vi "Initialize.vi"(8 "error in (no error)":errorcluster) -> (0 "error out":errorcluster, 3 "Available motors out":refnum<class "Motor-assembly.lvclass">)   [LabVIEW 2013, in "PowderDeposition.lvlib" / "Motor-assembly.lvclass"]
doc: "Create all motor objects and set the default settings contained in the 'Create' override of each specific motor class."
uses:
  Motor-assembly.lvclass
  Motor/Motor-Serial/Motor-Maxon/Motor-Zaxis/Motor-Zaxis.lvclass
  Motor/Motor-Serial/Motor-Maxon/Motor-Xaxis/Motor-Xaxis.lvclass
  Motor/Motor-Serial/Motor-GWInstek/Motor-Roller2/Motor-Roller2.lvclass
  Motor/Motor-Serial/Motor-GWInstek/Motor-Sieve2/Motor-Sieve2.lvclass
  Motor-assembly.lvclass/Motor-assembly.ctl
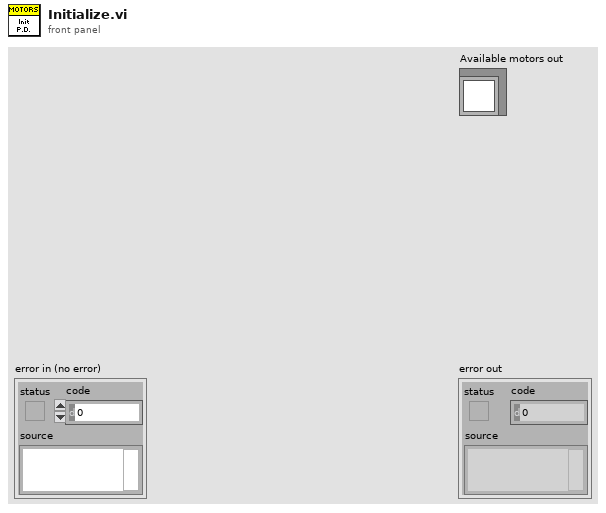
[diagram p1: front panel]
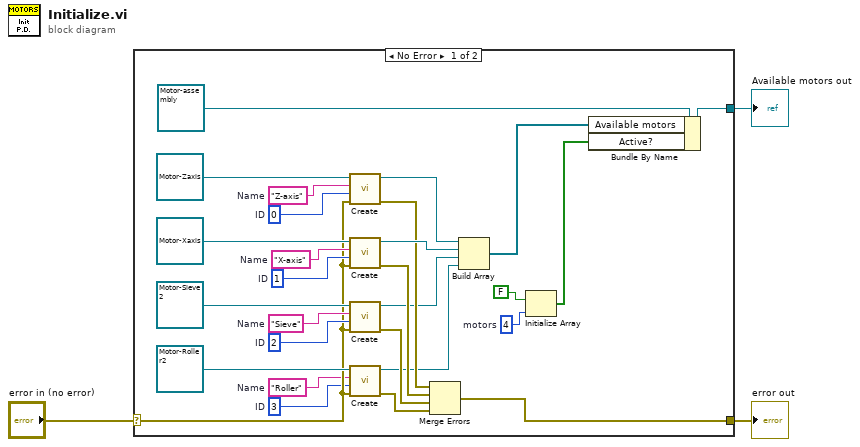
[diagram p0: block diagram]
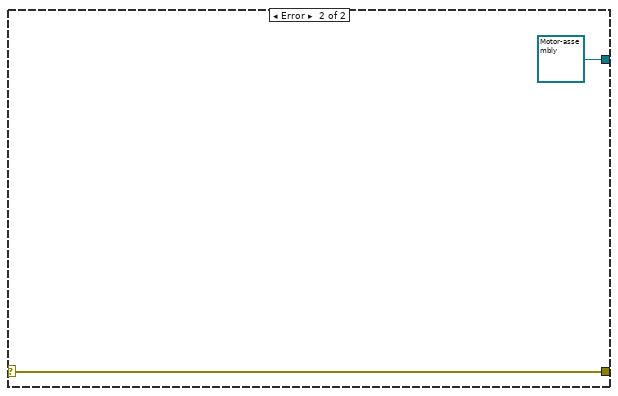
[diagram p2: hidden frame]
diagram:
  n1 = case shown="No Error" "error in (no error)" {
    selector: "error in (no error)" -> [w6 w33]
    tunnel: [w15 w33] -> w2
    tunnel: [w30 refnum<class "Motor-assembly.lvclass"> refnum ("Available motors in")] -> w1
    frame No Error {
      w20 = 4  # motors
      w5 = 3  # ID
      w4 = "Roller"  # Name
      w12 = 2  # ID
      w13 = "Sieve"  # Name
      w24 = 1  # ID
      w25 = "X-axis"  # Name
      w26 = 0  # ID
      w27 = "Z-axis"  # Name
      n2 = call-dynamic "Create.vi"("error in (no error)"=w6, "ID"=w26, "Name"=w27, "Motor in"=refnum<class "Motor-Zaxis.lvclass"> refnum ("Motor-Zaxis.lvclass")) -> ("error out"=w17:errorcluster, "Motor out"=w23:refnum<class "Motor-Zaxis.lvclass">)  [unwired: 6 in]
      n3 = call-dynamic "Create.vi"("error in (no error)"=w6, "ID"=w24, "Name"=w25, "Motor in"=refnum<class "Motor-Xaxis.lvclass"> refnum ("Motor-Xaxis.lvclass")) -> ("error out"=w16:errorcluster, "Motor out"=w22:refnum<class "Motor-Xaxis.lvclass">)  [unwired: 6 in]
      n4 = call-dynamic "Create.vi"("error in (no error)"=w6, "ID"=w12, "Name"=w13, "Motor in"=refnum<class "Motor-Sieve2.lvclass"> refnum ("Motor-Sieve2.lvclass")) -> ("error out"=w11:errorcluster, "Motor out"=w10:refnum<class "Motor-Sieve2.lvclass">)  [unwired: 6 in]
      n5 = call-dynamic "Create.vi"("error in (no error)"=w6, "ID"=w5, "Name"=w4, "Motor in"=refnum<class "Motor-Roller2.lvclass"> refnum ("Motor-Roller2.lvclass")) -> ("error out"=w7:errorcluster, "Motor out"=w8:refnum<class "Motor-Roller2.lvclass">)  [unwired: 6 in]
      n6 = Merge Errors(w17, w16, w11, w7) -> (w15:errorcluster)
      n7 = Build Array(w23, w22, w10, w8) -> (w19:refnum<class "Motor-Serial.lvclass">[])
      n8 = Initialize Array(FALSE, w20) -> (w18:bool[])
      n9 = Bundle By Name(cluster=refnum<class "Motor-assembly.lvclass"> refnum ("Available motors in"), "Available motors"=w19, "Active?"=w18) -> (w30:refnum<class "Motor-assembly.lvclass">)
    }
    frame Error {
    }
  }
  "error out" <- w2
  "Available motors out" <- w1
